vi "Compile Template.vi"(7 "Data":refnum<class "Datum.lvclass">=refnum, 8 "Error In":errorcluster, 10 "Output":path=path "", 11 "Template File Name":string) -> (0 "Error Out":errorcluster)   [LabVIEW 2018, in "Scripts.lvlib"]
uses:
  Scripts.lvlib
  Toolkit/Data/Datum/Datum.lvclass
  Toolkit/Data/Map/Map.lvclass
  Toolkit/Data/String/String.lvclass
  Toolkit/Support/Compile with Data.vi
  Toolkit/Toolkit.lvlib
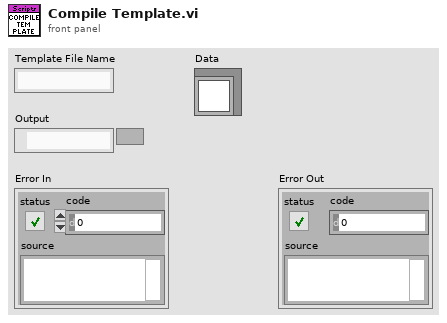
[diagram p1: front panel]
types:
  T1 = enum16{"open", "replace", "create", "open or create", "replace or create", "replace or create with confirmation"}
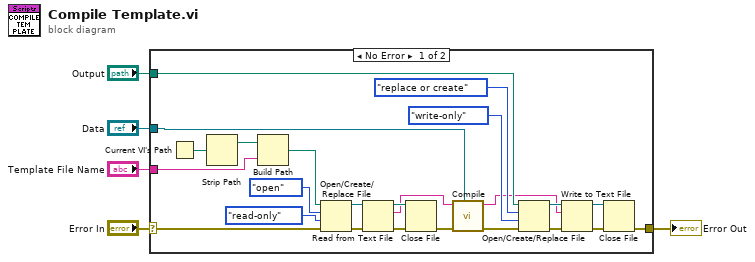
[diagram p0: block diagram]
diagram:
  n1 = case shown="No Error" "Error In" {
    selector: "Error In" -> [w10 w30]
    tunnel: "Output" -> [w20 _]
    tunnel: [w12 w30] -> w4
    tunnel: "Data" -> [w11 _]
    tunnel: "Template File Name" -> [w6 _]
    frame No Error {
      n2 = Current VI's Path() -> (path=w9:path)
      n3 = Strip Path(path=w9) -> (stripped path=w8:path)  [unwired: 1 out]
      n4 = Build Path(base path=w8, name or relative path=w6) -> (appended path=w7:path)
      n5 = Open/Create/Replace File(file path (use dialog)=w7, error in=w10, operation (0:open)=T1."open", access (0:read/write)=enum16{"read/write", "read-only", "write-only"}."read-only") -> (refnum out=w27:refnum<file>, error out=w26:errorcluster)  [unwired: 2 in, 1 out]
      n6 = Read from Text File(file (use dialog)=w27, error in=w26) -> (refnum out=w25:refnum<file>, text=w22:string, error out=w24:errorcluster)  [unwired: 2 in, 1 out]
      n7 = Close File(refnum=w25, error in=w24) -> (error out=w23:errorcluster)  [unwired: 1 out]
      n8 = call-poly "Compile.vi"("Data"=w11, "Error In"=w23, "Input"=w22) -> ("Error Out"=w21:errorcluster, "Output"=w15:string)  [unwired: 7 in]
      n9 = Open/Create/Replace File(file path (use dialog)=w20, error in=w21, operation (0:open)=T1."replace or create", access (0:read/write)=enum16{"read/write", "read-only", "write-only"}."write-only") -> (refnum out=w17:refnum<file>, error out=w16:errorcluster)  [unwired: 2 in, 1 out]
      n10 = Write to Text File(file (use dialog)=w17, text=w15, error in=w16) -> (refnum out=w14:refnum<file>, error out=w13:errorcluster)  [unwired: 1 in, 1 out]
      n11 = Close File(refnum=w14, error in=w13) -> (error out=w12:errorcluster)  [unwired: 1 out]
    }
    frame Error {
    }
  }
  "Error Out" <- w4
